vi "Emballage_fichierSpecifique_v2.vi"(5 "Indice Rev. Client":string, 7 "N° article client":string, 8 "error in (no error)":errorcluster caption="entrée d'erreur (pas d'erreur)", 10 "Tableau n° valves":string[](array[string])=["100200021121130326", "100200021121130308", "100200021121130314", "100200021121130316", "100200021121130319", "100200021121130330", "100200021121130309", "100200021121130307", "100200021121130311", "100200021121130299", "100200021121130310", "100200021121130313", "100200021121130321", "100200021121130336", "100200021121130322", "100200021121130302", "100200021121130334", "100200021121130317", "100200021121130348", "100200021121130333", "100200021121130355", "100200021121130345", "100200021121130349", "100200021121130350", "100200021121130315", "100200021121130352", "100200021121130328", "100200021121130337", "100200021121130357", "100200021121130359", "100200021121130360", "100200021121130344", "100200021121130347", "100200021121130358", "100200021121130341", "100200021121130338", "100200021121130331", "100200021121130329", "100200021121130332", "100200021121130339", "100200021121130340", "100200021121130343", "100200021121130351", "100200021121130354", "100200021121130346", "100200021121130335", "100200021121130342", "100200021121130353", "100200021121130383", "100200021121130384", "100200021121130380", "100200021121130389", "100200021121130382", "100200021121130379", "100200021121130376", "100200021121130378", "100200021121130391", "100200021121130392", "100200021121130372", "100200021121130362", "100200021121130375", "100200021121130371", "100200021121130385", "100200021121130364", "100200021121130386", "100200021121130361", "100200021121130366", "100200021121130365", "100200021121130367", "100200021121130363", "100200021121130377", "100200021121130374", "100200021121130369", "100200021121130370", "100200021121130373", "100200021121130388", "100200021121130368", "100200021121130356", "100200021121130412", "100200021121130407", "100200021121130406", "100200021121130408", "100200021121130398", "100200021121130415", "100200021121130402", "100200021121130399", "100200021121130414", "100200021121130413", "100200021121130393", "100200021121130390", "100200021121130403", "100200021121130401", "100200021121130387", "100200021121130381", "100200021121130395", "100200021121130394", "100200021121130411", "100200021121130410", "100200021121130405", "100200021121130396", "100200021121130397", "100200021121130400", "100200021121130404", "100200021121130211", "100200021121130215", "100200021121130217", "100200021121130212", "100200021121130219", "100200021121130225", "100200021121130213", "100200021121130216", "100200021121130226", "100200021121130224", "100200021121130223", "100200021121130230", "100200021121130220", "100200021121130214", "100200021121130229", "100200021121130236", "100200021121130238", "100200021121130239", "100200021121130237", "100200021121130234", "100200021121130242", "100200021121130241", "100200021121130233", "100200021121130210", "100200021121130218", "100200021121130240", "100200021121130221", "100200021121130245", "100200021121130222", "100200021121130235", "100200021121130247", "100200021121130227", "100200021121130231", "100200021121130228", "100200021121130243", "100200021121130246", "100200021121130251", "100200021121130273", "100200021121130267", "100200021121130268", "100200021121130256", "100200021121130265", "100200021121130261", "100200021121130264", "100200021121130254", "100200021121130257", "100200021121130249", "100200021121130248", "100200021121130250", "100200021121130244", "100200021121130253", "100200021121130266", "100200021121130252", "100200021121130274", "100200021121130263", "100200021121130232", "100200021121130262", "100200021121130260", "100200021121130269", "100200021121130270", "100200021121130294", "100200021121130255", "100200021121130258", "100200021121130295", "100200021121130297", "100200021121130291", "100200021121130289", "100200021121130278", "100200021121130283", "100200021121130284", "100200021121130296", "100200021121130277", "100200021121130286", "100200021121130288", "100200021121130287", "100200021121130275", "100200021121130290", "100200021121130298", "100200021121130279", "100200021121130292", "100200021121130259", "100200021121130293", "100200021121130272", "100200021121130271", "100200021121130276", "100200021121130282", "100200021121130281", "100200021121130280", "100200021121130285", "100200021121130300", "100200021121130152", "100200021121130165", "100200021121130178", "100200021121130151", "100200021121130175", "100200021121130173", "100200021121130157", "100200021121130167", "100200021121130155", "100200021121130174", "100200021121130164", "100200021121130163", "100200021121130159", "100200021121130160", "100200021121130186", "100200021121130154", "100200021121130169", "100200021121130166", "100200021121130156", "100200021121130207", "100200021121130192", "100200021121130158", "100200021121130161", "100200021121130168", "100200021121130170", "100200021121130171", "100200021121130162", "100200021121130190", "100200021121130191", "100200021121130193", "100200021121130182", "100200021121130183", "100200021121130176", "100200021121130148", "100200021121130177", "100200021121130203", "100200021121130184", "100200021121130189", "100200021121130194", "100200021121130179", "100200021121130196", "100200021121130188", "100200021121130180", "100200021121130187", "100200021121130181", "100200021121130195", "100200021121130185", "100200021121130204", "100200021121130202", "100200021121130200", "100200021121130198", "100200021121130197", "100200021121130199", "100200021121130150", "100200021121130111", "100200021121130201", "100200021121130208", "100200021121130209", "100200021121130205", "100200021121130206", "100200021121130093", "100200021121130091", "100200021121130109", "100200021121130088", "100200021121130099", "100200021121130097", "100200021121130096", "100200021121130102", "100200021121130095", "100200021121130092", "100200021121130094", "100200021121130098", "100200021121130101", "100200021121130100", "100200021121130106", "100200021121130121", "100200021121130104", "100200021121130107", "100200021121130089", "100200021121130103", "100200021121130105", "100200021121130108", "100200021121130120", "100200021121130125", "100200021121130138", "100200021121130114", "100200021121130115", "100200021121130119", "100200021121130118", "100200021121130117", "100200021121130113", "100200021121130112", "100200021121130124", "100200021121130110", "100200021121130116", "100200021121130149", "100200021121130145", "100200021121130127", "100200021121130130", "100200021121130128", "100200021121130129", "100200021121130134", "100200021121130133", "100200021121130135", "100200021121130143", "100200021121130139", "100200021121130147", "100200021121130136", "100200021121130141", "100200021121130144", "100200021121130126", "100200021121130123", "100200021121130122", "100200021121130132", "100200021121130131", "100200021121130140", "100200021121130146", "100200021121130137", "100200021121130142", "100200021121130153", "100200021121130060", "100200021121130077", "100200021121130059", "100200021121130040", "100200021121130075", "100200021121130082", "100200021121130022", "100200021121130086", "100200021121130045", "100200021121130078", "100200021121130080", "100200021121130074", "100200021121130065", "100200021121130066", "100200021121130070", "100200021121130068", "100200021121130084", "100200021121130069", "100200021121130076", "100200021121130081", "100200021121130083", "100200021121130085", "100200021121130087", "100200021121130090", "100200021121130012", "100200021121130028", "100200021121130079", "100200021121130073", "100200021121130072", "100200021121130071", "100200021121130042", "100200021121130030", "100200021121130033", "100200021121130032", "100200021121130027", "100200021121130031", "100200021121130025", "100200021121130020", "100200021121130026", "100200021121130003", "100200021121130008", "100200021121130001", "100200021121130019", "100200021121120509", "100200021121130021", "100200021121130016", "100200021121130013", "100200021121120510", "100200021121130015", "100200021121130002", "100200021121130014", "100200021121130029", "100200021121130049", "100200021121130048", "100200021121130011", "100200021121130063", "100200021121130009", "100200021121130010", "100200021121130004", "100200021121130017", "100200021121130018", "100200021121130024", "100200021121130023", "100200021121130061", "100200021121130062", "100200021121130064", "100200021121130058", "100200021121130046", "100200021121130056", "100200021121130057", "100200021121130054", "100200021121130051", "100200021121130044", "100200021121130035", "100200021121130043", "100200021121130005", "100200021121130038", "100200021121130039", "100200021121130047", "100200021121130053", "100200021121130007", "100200021121130037", "100200021121130006", "100200021121130052", "100200021121130041", "100200021121130034", "100200021121130036", "100200021121130067", "100200021121130050", "100200021121130055", "100200021121120410", "100200021121120406", "100200021121120421", "100200021121120408", "100200021121120424", "100200021121120416", "100200021121120423", "100200021121120419", "100200021121120407", "100200021121120397", "100200021121120396", "100200021121120404", "100200021121120422", "100200021121120392", "100200021121120403", "100200021121120405", "100200021121120400", "100200021121120385", "100200021121120348", "100200021121120388", "100200021121120414", "100200021121120412", "100200021121120320", "100200021121120394", "100200021121120447", "100200021121120398", "100200021121120444", "100200021121120417", "100200021121120395", "100200021121120402", "100200021121120401", "100200021121120393", "100200021121120399", "100200021121120425", "100200021121120449", "100200021121120415", "100200021121120446", "100200021121120439", "100200021121120426", "100200021121120434", "100200021121120453", "100200021121120455", "100200021121120441", "100200021121120443", "100200021121120435", "100200021121120409", "100200021121120420", "100200021121120427", "100200021121120429", "100200021121120438", "100200021121120432", "100200021121120437", "100200021121120430", "100200021121120440", "100200021121120442", "100200021121120428", "100200021121120464", "100200021121120433", "100200021121120418", "100200021121120445", "100200021121120431", "100200021121120463", "100200021121120451", "100200021121120466", "100200021121120454", "100200021121120452", "100200021121120459", "100200021121120411", "100200021121120458", "100200021121120472", "100200021121120470", "100200021121120474", "100200021121120462", "100200021121120477", "100200021121120436", "100200021121120469", "100200021121120467", "100200021121120413", "100200021121120460", "100200021121120486", "100200021121120476", "100200021121120473", "100200021121120468", "100200021121120478", "100200021121120482", "100200021121120471", "100200021121120479", "100200021121120456", "100200021121120465", "100200021121120461", "100200021121120488", "100200021121120457", "100200021121120475", "100200021121120489", "100200021121120493", "100200021121120487", "100200021121120485"], 11 "Datetime":string="06.04.2021 15:16:41") -> (0 "error out":errorcluster caption="sortie d'erreur")   [LabVIEW 2020]
uses:
  Modules/FS/60_FS_Controles/60_FS_SetGet.ctl
  <vilib>/Utility/NIReport.llb/NI_report.lvclass
  <vilib>/Utility/NIReport.llb/Report Type.ctl
  <vilib>/Utility/NIReport.llb/NI_ReportGenerationCore.lvlib
  <vilib>/Utility/NIReport.llb/Excel/NI_Excel.lvclass
  <vilib>/Utility/NIReport.llb/Append Text Table to Report (wrap).vi
panel:
  out "All Files in Dir 2":path[](array[path]) caption="Tous les fichiers du rép."
  out "Number of Files 2":i32 caption="Nombre de fichiers"
  out "path out":path
  out "IsSuccessful":bool
  in  "appended path":path=path "C:/Users/ltinguely/Documents"
  out "chaîne résultante":string
  out "Number of Files":i32 caption="Nombre de fichiers"
  out "All Files in Dir":path[](array[path]) caption="Tous les fichiers du rép."
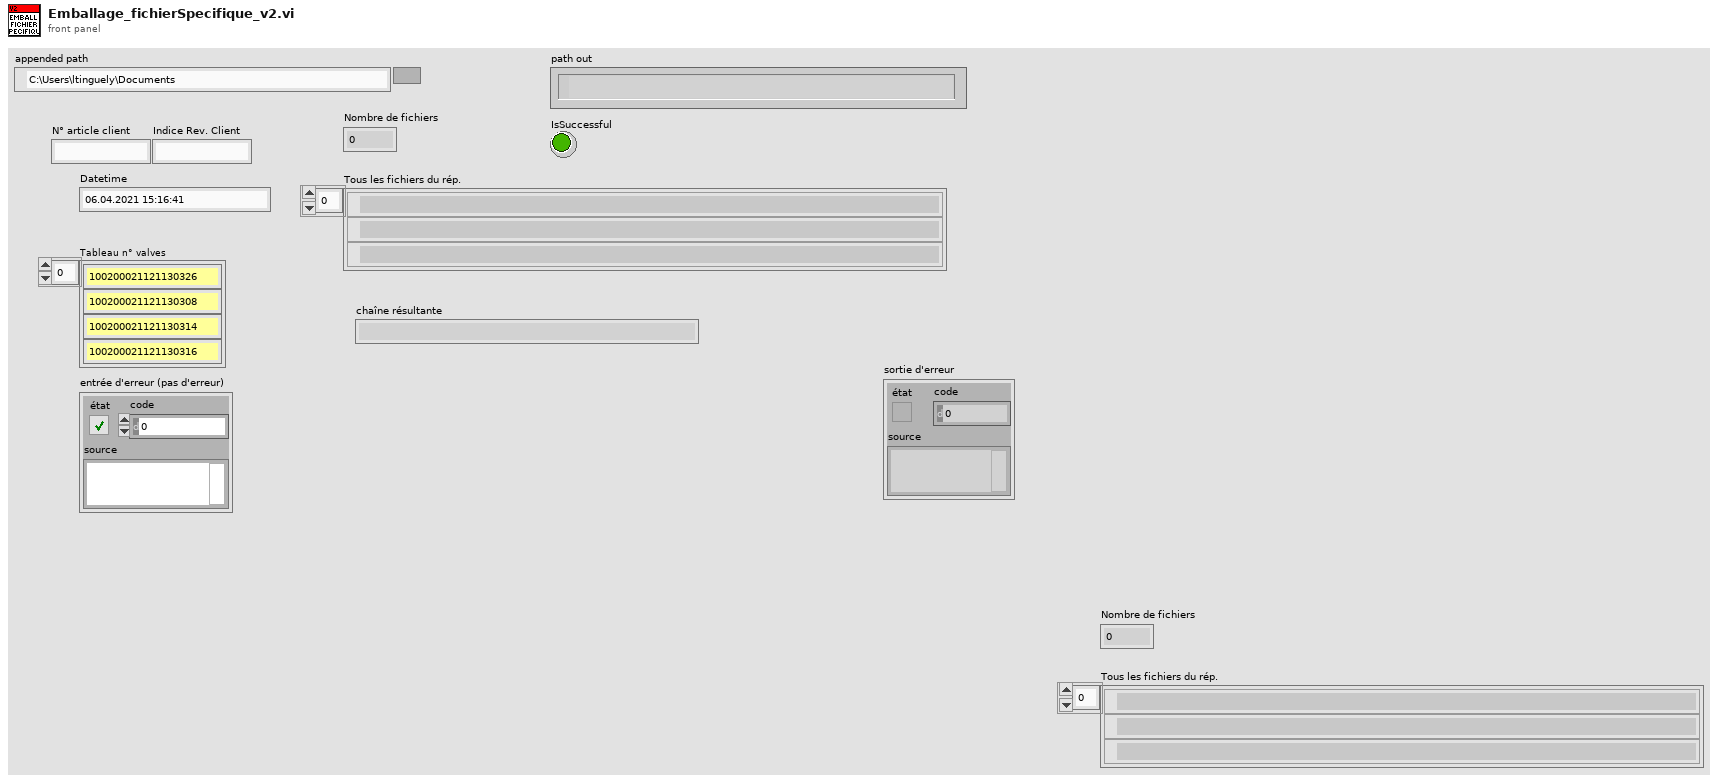
[diagram p1: front panel]
types:
  T1 = typedef "60_FS_SetGet.ctl" = enum16{"set", "get"}
  T2 = cluster{"position (Excel)":cluster{"row":i32, "column":i32}, "name (Excel)":string, "bookmark (Word)":string}
  T3 = typedef "NI_ReportGenerationCore.lvlib/Report Type.ctl" = enum16{"HTML", "Word", "Excel"}
  T4 = typedef "60_FS_CLT_Chemins.ctl" = cluster{"Racine_local":path, "Racine_reseau":path, "Racine_Support_Application":path, "Fichier_Journalisation":path, "Connexion_BDD_VSX":path, "Connexion_BDD_PLZ":path}
  T5 = typedef "Emballage_BDD_param_Produit.ctl" = cluster{"No_Valve_FAS":string, "suffixe":string, "designation":string, "indice_produit":string, "code_barre_fixe":string, "affiche_code_barre_client":string, "affiche_no_client":string, "Nb_vlve_par_carton":u16, "melange_des_lots_possible":string, "id_article":string, "Indice_Rev":string, "Famille":string, "date":string, "code_barre_fixe_Fin":string, "Longeur_No_Serie":string}
  T6 = cluster{"on/off":bool, "weight":i32, "color":u32}
  T7 = cluster{"start (wd) - row (xl) ":i32, "end (wd) - col (xl) ":i32}
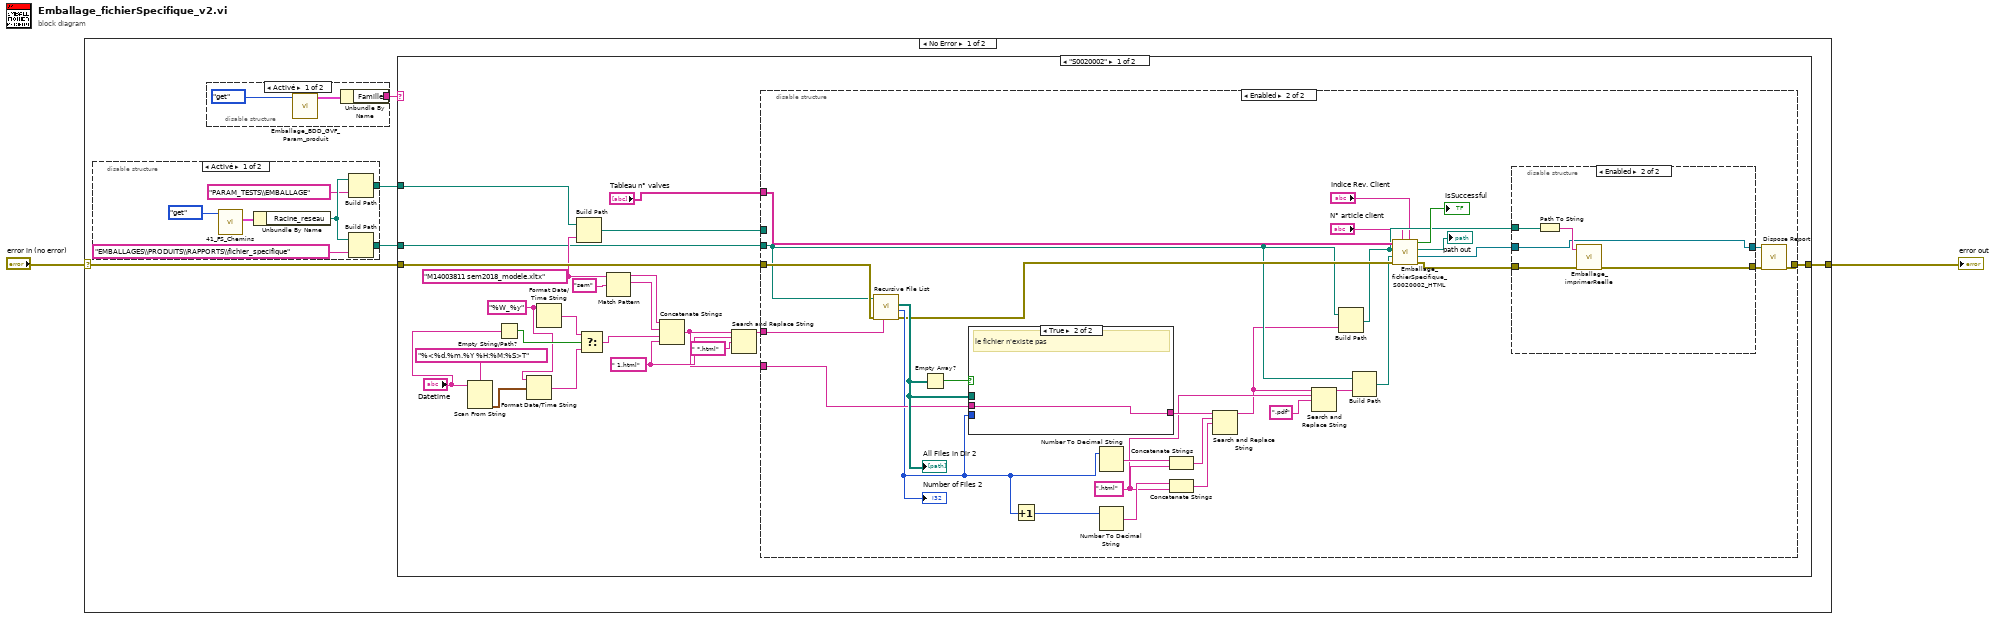
[diagram p0: block diagram]
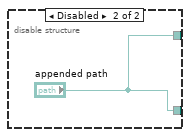
[diagram p2: hidden frame]
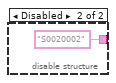
[diagram p3: hidden frame]
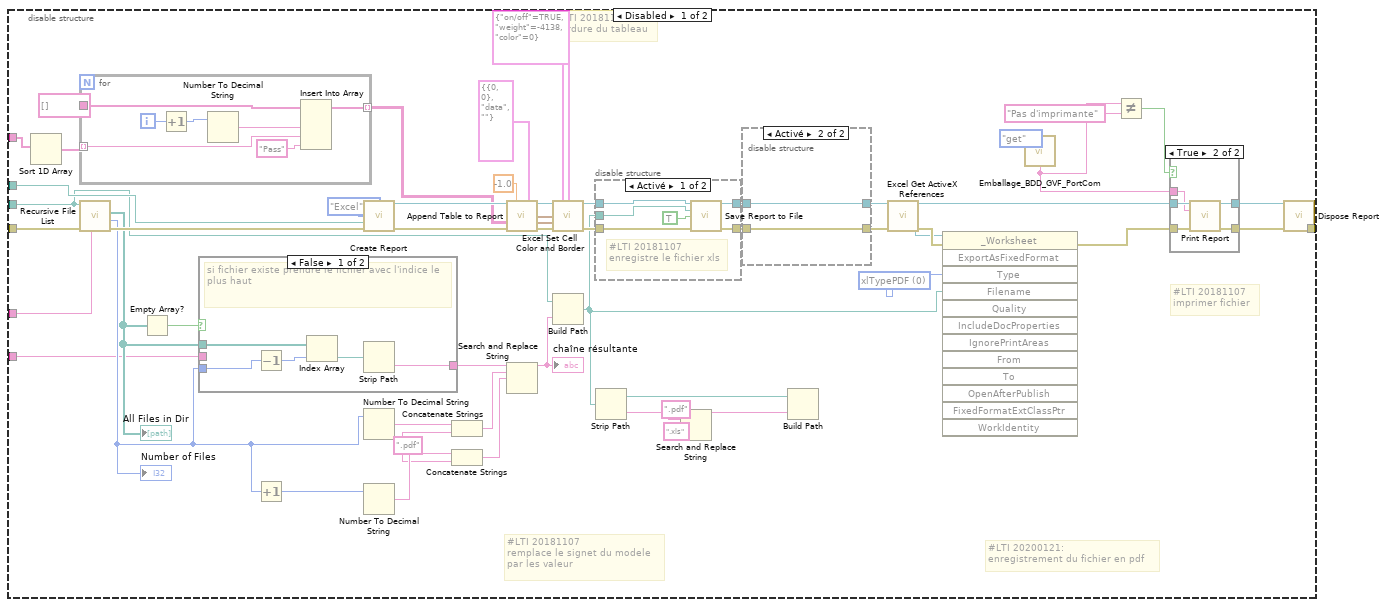
[diagram p4: hidden frame]
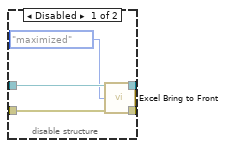
[diagram p5: hidden frame]
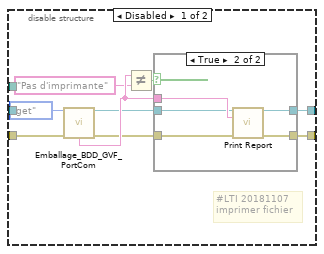
[diagram p9: hidden frame]
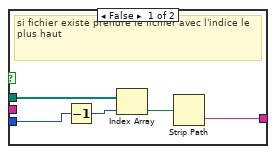
[diagram p11: hidden frame]
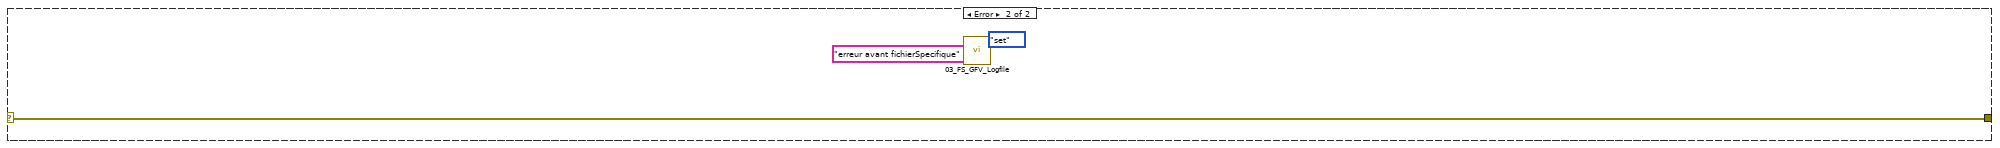
[diagram p13: hidden frame]
diagram:
  n1 = case shown="No Error" "error in (no error)" {
    selector: "error in (no error)" -> [w5 w190]
    tunnel: [w7 w190] -> w1
    frame No Error {
      n2 = disable-structure shown="Activé" {
        disable-tunnel: [w10 "appended path"] -> w4
        disable-tunnel: [w8 "appended path"] -> w3
        frame Enabled {
          n3 = call "41_FS_Chemins.vi"("SetGet"=60_FS_SetGet."get") -> ("CLT_Chemins_out"=w14:T4)  [unwired: 9 in, 1 out]
          n4 = Unbundle By Name(w14) -> ("Racine_reseau"=w11:path)
          n5 = Build Path(base path=w11, name or relative path="PARAM_TESTS\\EMBALLAGE" ("nom ou chemin relatif")) -> (appended path=w10:path)
          n6 = Build Path(base path=w11, name or relative path="EMBALLAGES\\PRODUITS\\RAPPORTS\\fichier_specifique" ("nom ou chemin relatif")) -> (appended path=w8:path)
        }
        frame Disabled {
        }
      }
      n7 = disable-structure shown="Activé" {
        disable-tunnel: [w16 "S0020002" ("Famille")] -> w6
        frame Enabled {
          n8 = call "Emballage_BDD_GVF_Param_produit.vi"("Énum"=enum16{"set", "get"}."get") -> ("CLS_param_produit"=w17:T5)  [unwired: 7 in, 3 out]
          n9 = Unbundle By Name(w17) -> ("Famille"=w16:string)
        }
        frame Disabled {
        }
      }
      n10 = case shown="\"S0020002\"" w6 {
        tunnel: w4 -> [w41 _]
        tunnel: w5 -> [w35 w189]
        tunnel: [w31 w189] -> w7
        tunnel: w3 -> [w29 _]
        frame "S0020002" {
          w30 = "M14003811 sem2018_modele.xltx"
          w34 = " 1.html" ("chaîne")
          w21 = "%W_%y" ("chaîne de format de l'heure (%c)")
          n11 = Scan From String(format string="%<%d.%m.%Y %H:%M:%S>T" ("chaîne de format"), input string="Datetime") -> (output 1=w23:timestamp)  [unwired: 3 in, 3 out]
          n12 = Empty String/Path?(string/path="Datetime") -> (empty?=w26:bool)
          n13 = Format Date/Time String(time format string (%c)=w21, seconds (now)=w23) -> (date/time string=w22:string)  [unwired: 1 in]
          n14 = Format Date/Time String(time format string (%c)=w21) -> (date/time string=w25:string)  [unwired: 2 in]
          n15 = Build Path(base path=w41, name or relative path=w30) -> (appended path=w40:path)
          n16 = Select(t=w25, s=w26, f=w22) -> (s? t:f=w24:string)
          n17 = Match Pattern(string=w30, regular expression="sem" ("expression régulière")) -> (before substring=w39:string, match substring=w37:string)  [unwired: 1 in, 2 out]
          n18 = Concatenate Strings(w39, w37, w24, w34) -> (w32:string)
          n19 = Search and Replace String(input string=w32, search string=w34, replace string=" *.html" ("chaîne de remplacement (\"\")")) -> (result string=w33:string)  [unwired: 5 in, 3 out]
          n20 = disable-structure shown="Enabled" {
            disable-tunnel: w40 -> [w89 _]
            disable-tunnel: w35 -> [w88 w152]
            disable-tunnel: w33 -> [w75 w150]
            disable-tunnel: w32 -> [w74 w149]
            disable-tunnel: [w73 w142] -> w31
            disable-tunnel: w29 -> [w63 w138]
            disable-tunnel: "Tableau n° valves" -> [w43 w161]
            frame Disabled {
              w51 = 0 items=["xlTypePDF", "xlTypeXPS"] ("Type")
              w81 = ".pdf" ("chaîne")
              w64 = T6 {"on/off"=TRUE, "weight"=-4138, "color"=0} ("outside border")
              # "#LTI 20200121:\nenregistrement du fichier en pdf"
              # "#LTI 20181107\nimprimer fichier"
              # "#LTI 20181107\nbordure du tableau"
              # "#LTI 20181107\nremplace le signet du modele\npar les valeur"
              n21 = Sort 1D Array(array=w43) -> (sorted array=w42:string[])
              n22 = for {
                tunnel: w42 -> [w121] mode=indexing
                tunnel: string[] [] -> [w125]
                tunnel: [w119] -> w71 mode=indexing
                i -> [w124]
                n23 = Increment(x=w124) -> (x+1=w123:i32)
                n24 = Number To Decimal String(number=w123) -> (decimal integer string=w122:string)  [unwired: 1 in]
                n25 = Insert Into Array(array=w125, new element #1=w122, new element #2=w121, new element #3="Pass" ("nouvel élément/sous-tableau")) -> (w119:string[])  [unwired: 1 in]
              }
              n26 = call <vilib>:"Recursive File List.vi"("pattern"=w75, "error in (no error)"=w88, "Folder Path"=w63) -> ("error out"=w87:errorcluster, "Number of Files"=w79:i32, "All Files in Dir"=w77:path[])  [unwired: 4 in, 2 out]
              "Number of Files" <- w79
              "All Files in Dir" <- w77
              n27 = Empty Array?(array=w77) -> (empty?=w78:bool)
              n28 = case shown="False" w78 {
                tunnel: w77 -> [w130 _]
                tunnel: w79 -> [w128 _]
                tunnel: [w126 w131] -> w76
                tunnel: w74 -> [_ w131]
                frame False {
                  # "si fichier existe prendre le fichier avec l'indice le plus haut"
                  n29 = Decrement(x=w128) -> (x-1=w129:i32)
                  n30 = Index Array(array=w130, index=w129) -> (element=w127:path)
                  n31 = Strip Path(path=w127) -> (name=w126:string)  [unwired: 1 out]
                }
                frame True {
                  # "le fichier n'existe pas"
                }
              }
              n32 = Increment(x=w79) -> (x+1=w85:i32)
              n33 = call <vilib>:"Create Report.vi"("report type"=Report_Type."Excel" ("Report Type"), "template (empty)"=w89, "error in (no error)"=w87) -> ("report out"=w93:refnum<class "NI_report.lvclass">, "error out"=w94:errorcluster)  [unwired: 11 in]
              n34 = Number To Decimal String(number=w79) -> (decimal integer string=w84:string)  [unwired: 1 in]
              n35 = Number To Decimal String(number=w85) -> (decimal integer string=w86:string)  [unwired: 1 in]
              n36 = Concatenate Strings(w84, w81) -> (w83:string)
              n37 = Concatenate Strings(w86, w81) -> (w82:string)
              n38 = call-poly <vilib>:"Append Table to Report.vi"("report in"=w93, "column width (1)"=-1.0, "MS Office parameters"=T2 {"position (Excel)"={"row"=0, "column"=0}, "name (Excel)"="data", "bookmark (Word)"=""}, "text data"=w71, "error in (no error)"=w94) -> ("report out"=w68:refnum<class "NI_report.lvclass">, "range (wd) - start (xl)"=w70:T7, "end (xl)"=w69:cluster{"row (xl) ":i32, "col (xl) ":i32}, "error out"=w66:errorcluster)  [unwired: 7 in]
              n39 = Search and Replace String(input string=w76, search string=w83, replace string=w82) -> (result string=w80:string)  [unwired: 5 in, 3 out]
              "chaîne résultante" <- w80
              n40 = call <vilib>:"Excel Set Cell Color and Border.vi"("report in"=w68, "inside border"=w64, "outside border"=w64, "start (-1, -1)"=w70, "end (-1, -1)"=w69, "error in (no error)"=w66) -> ("report out"=w67:refnum<class "NI_report.lvclass">, "error out"=w65:errorcluster)  [unwired: 8 in]
              n41 = Build Path(base path=w63, name or relative path=w80) -> (appended path=w44:path)
              n42 = disable-structure shown="Activé" {
                disable-tunnel: [w109 w111] -> w96
                disable-tunnel: [w108 w110] -> w95
                disable-tunnel: w44 -> [w106 _]
                disable-tunnel: w67 -> [w105 w110]
                disable-tunnel: w65 -> [w104 w111]
                frame Enabled {
                  # "#LTI 20181107\nenregistre le fichier xls"
                  n43 = call-dynamic "Save Report to File.vi"("report in"=w105, "report file path"=w106, "prompt to replace? (F)"=TRUE, "error in (no error)"=w104) -> ("report out"=w108:refnum<class "NI_report.lvclass">, "error out"=w109:errorcluster)  [unwired: 10 in]
                }
                frame Disabled {
                }
              }
              n44 = Strip Path(path=w44) -> (stripped path=w49:path, name=w48:string)
              n45 = Search and Replace String(input string=w48, search string=".pdf" ("chaîne de remplacement (\"\")"), replace string=".xls" ("chaîne recherchée")) -> (result string=w47:string)  [unwired: 5 in, 3 out]
              n46 = disable-structure shown="Activé" {
                disable-tunnel: w96 -> [w101 w102]
                disable-tunnel: w95 -> [w100 w103]
                disable-tunnel: [w98 w102] -> w62
                disable-tunnel: [w97 w103] -> w61
                frame Disabled {
                  n47 = call <vilib>:"Excel Bring to Front.vi"("report in"=w100, "window state (maximized)"=enum16{"maximized", "minimized", "normal"}."maximized", "error in (no error)"=w101) -> ("report out"=w97:refnum<class "NI_report.lvclass">, "error out"=w98:errorcluster)  [unwired: 11 in]
                }
                frame Enabled {
                }
              }
              n48 = Build Path(base path=w49, name or relative path=w47) -> ()  [unwired: 1 out]
              n49 = call <vilib>:"Excel Get ActiveX References.vi"("report in"=w61, "error in (no error)"=w62) -> ("report out"=w54:refnum<class "NI_report.lvclass">, "Excel._Worksheet"=w50:refnum<k7>, "error out"=w55:errorcluster)  [unwired: 7 in, 4 out]
              n50 = invoke class="_Worksheet" method="ExportAsFixedFormat"(reference=w50, error in=w55, "Type"=w51, "Filename"=w44) -> (error out=w60:errorcluster)  [unwired: 9 in, 12 out]
              n51 = call "Emballage_BDD_GVF_PortCom.vi"("Énum"=enum16{"get", "set"}."get") -> ("Imprimante Certif."=w58:string)  [unwired: 8 in, 6 out]
              n52 = Not Equal?(x=w58, y="Pas d'imprimante") -> (x != y?=w57:bool)
              n53 = case shown="True" w57 {
                tunnel: [w112 w118] -> w52
                tunnel: w54 -> [w113 w117]
                tunnel: [w113 w116] -> w53
                tunnel: w60 -> [w112 w115]
                tunnel: w58 -> [_ w114]
                frame False {
                }
                frame True {
                  n54 = call-dynamic "Print Report.vi"("report in"=w117, "printer name (default)"=w114, "error in (no error)"=w115) -> ("report out"=w116:refnum<class "NI_report.lvclass">, "error out"=w118:errorcluster)  [unwired: 11 in]
                }
              }
              n55 = call-dynamic "Dispose Report.vi"("report in"=w53, "error in (no error)"=w52) -> ("error out"=w73:errorcluster)  [unwired: 13 in]
            }
            frame Enabled {
              w146 = ".html" ("chaîne")
              n56 = call <vilib>:"Recursive File List.vi"("pattern"=w150, "error in (no error)"=w152, "Folder Path"=w138) -> ("error out"=w147:errorcluster, "Number of Files"=w148:i32, "All Files in Dir"=w151:path[])  [unwired: 4 in, 2 out]
              "Number of Files 2" <- w148
              "All Files in Dir 2" <- w151
              n57 = Empty Array?(array=w151) -> (empty?=w154:bool)
              n58 = case shown="True" w154 {
                tunnel: w151 -> [w187 _]
                tunnel: w148 -> [w185 _]
                tunnel: [w183 w188] -> w153
                tunnel: w149 -> [_ w188]
                frame False {
                  # "si fichier existe prendre le fichier avec l'indice le plus haut"
                  n59 = Decrement(x=w185) -> (x-1=w186:i32)
                  n60 = Index Array(array=w187, index=w186) -> (element=w184:path)
                  n61 = Strip Path(path=w184) -> (name=w183:string)  [unwired: 1 out]
                }
                frame True {
                  # "le fichier n'existe pas"
                }
              }
              n62 = Increment(x=w148) -> (x+1=w158:i32)
              n63 = Number To Decimal String(number=w148) -> (decimal integer string=w157:string)  [unwired: 1 in]
              n64 = Number To Decimal String(number=w158) -> (decimal integer string=w159:string)  [unwired: 1 in]
              n65 = Concatenate Strings(w157, w146) -> (w156:string)
              n66 = Concatenate Strings(w159, w146) -> (w155:string)
              n67 = Search and Replace String(input string=w153, search string=w156, replace string=w155) -> (result string=w137:string)  [unwired: 5 in, 3 out]
              n68 = Search and Replace String(input string=w137, search string=w146, replace string=".pdf" ("chaîne de remplacement (\"\")")) -> (result string=w139:string)  [unwired: 5 in, 3 out]
              n69 = Build Path(base path=w138, name or relative path=w137) -> (appended path=w134:path)
              n70 = Build Path(base path=w138, name or relative path=w139) -> (appended path=w136:path)
              n71 = call "Emballage_fichierSpecifique_S0020002_HTML.vi"("Indice Rev. Client"="Indice Rev. Client", "N° article client"="N° article client", "Error in"=w147, "PDF filename path"=w136, "report file path"=w134, "Tableau n° valves"=w161) -> ("Error out"=w135:errorcluster, "report out"=w144:refnum<class "NI_report.lvclass">, "path out"=→"path out":path, "IsSuccessful"=→"IsSuccessful":bool)  [unwired: 2 in]
              n72 = disable-structure shown="Enabled" {
                disable-tunnel: w144 -> [w166 w178]
                disable-tunnel: [w165 w181] -> w141
                disable-tunnel: [w164 w178] -> w140
                disable-tunnel: w135 -> [w163 w182]
                disable-tunnel: w134 -> [_ w180]
                frame Disabled {
                  # "#LTI 20181107\nimprimer fichier"
                  n73 = call "Emballage_BDD_GVF_PortCom.vi"("Énum"=enum16{"get", "set"}."get", "Error in"=w163) -> ("Imprimante Certif."=w169:string, "Error out"=w162:errorcluster)  [unwired: 7 in, 5 out]
                  n74 = Not Equal?(x=w169, y="Pas d'imprimante") -> (x != y?=w170:bool)
                  n75 = case shown="True" w170 {
                    tunnel: [w171 w177] -> w165
                    tunnel: w166 -> [w172 w175]
                    tunnel: [w172 w174] -> w164
                    tunnel: w162 -> [w171 w173]
                    tunnel: w169 -> [_ w176]
                    frame False {
                    }
                    frame True {
                      n76 = call-dynamic "Print Report.vi"("report in"=w175, "printer name (default)"=w176, "error in (no error)"=w173) -> ("report out"=w174:refnum<class "NI_report.lvclass">, "error out"=w177:errorcluster)  [unwired: 11 in]
                    }
                  }
                }
                frame Enabled {
                  n77 = Path To String(path=w180) -> (string=w179:string)
                  n78 = call "Emballage_imprimerReelle.vi"("path to HTML"=w179, "Error in"=w182) -> ("sortie d'erreur"=w181:errorcluster)  [unwired: 8 in]
                }
              }
              n79 = call-dynamic "Dispose Report.vi"("report in"=w140, "error in (no error)"=w141) -> ("error out"=w142:errorcluster)  [unwired: 13 in]
            }
          }
        }
        frame "", Default {
          # "pas de fichier spécifique pour le produit sélectionné"
        }
      }
    }
    frame Error {
      n80 = call "03_FS_GFV_Logfile.vi"("Chaîne"="erreur avant fichierSpecifique", "States"=60_FS_SetGet."set") -> ()  [unwired: 8 in, 2 out]
    }
  }
  "error out" <- w1
